vi "Get_from_WebActivex.vi"() -> ()   [LabVIEW 2016]
panel:
  out "lVideoWindNum":i32
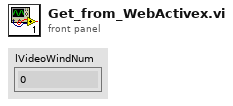
[diagram p1: front panel]
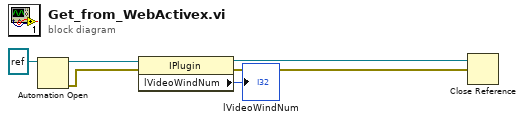
[diagram p0: block diagram]
diagram:
  n1 = Automation Open(Automation Refnum=refnum<k7> refnum ("WEBACTIVEXLib.IPlugin")) -> (Automation Refnum=w4:refnum<k7>, error out=w5:errorcluster)  [unwired: 3 in]
  n2 = property class="IPlugin"(reference=w4, error in=w5) -> (reference out=w3:refnum<k7>, error out=w2:errorcluster, "lVideoWindNum"=→"lVideoWindNum":i32)
  n3 = Close Reference(reference=w3, error in (no error)=w2) -> ()  [unwired: 1 out]
